vi "Data.vi"(8 "error in":errorcluster, 10 "Исходные данные":T1) -> (0 "error out":errorcluster)   [LabVIEW 2023, in "Initial Data.lvlib"]
doc: "_____\nCreated using DQMH Event Scripter 6.1.0.128."
uses:
  Initial Data.lvlib
  InitalData Type.ctl
  Data Argument--cluster.ctl
panel:
  # "Образец"
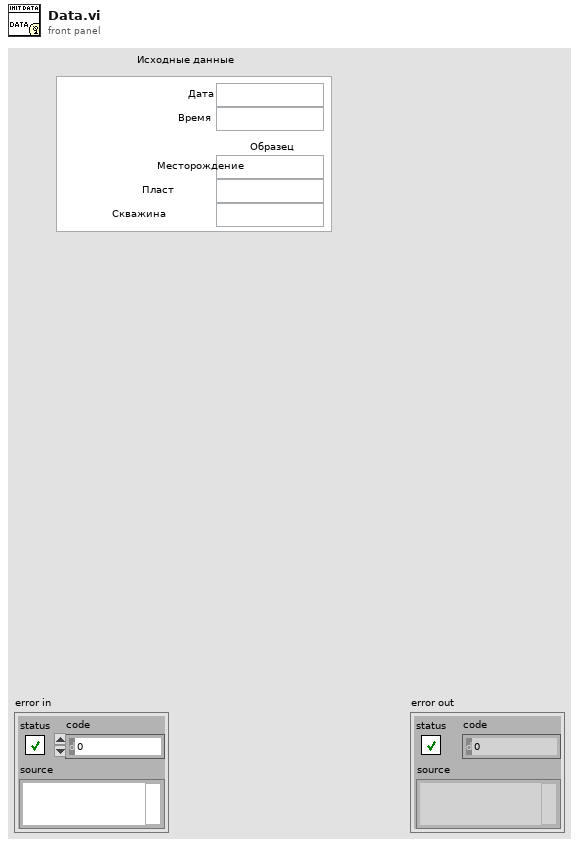
[diagram p1: front panel]
types:
  T1 = typedef "Initial Data.lvlib/InitalData Type.ctl" = cluster{"Дата":string, "Время":string, "Месторождение":string, "Пласт":string, "Скважина":string}
  T2 = typedef "Initial Data.lvlib/Data Argument--cluster.ctl" = cluster{"Исходные данные":T1}
  T3 = typedef "Initial Data.lvlib/Broadcast Events--cluster.ctl" = cluster{"Module Did Init":refnum<user-event>, "Status Updated":refnum<user-event>, "Error Reported":refnum<user-event>, "Module Did Stop":refnum<user-event>, "Update Module Execution Status":refnum<user-event>, "Data":refnum<user-event>}
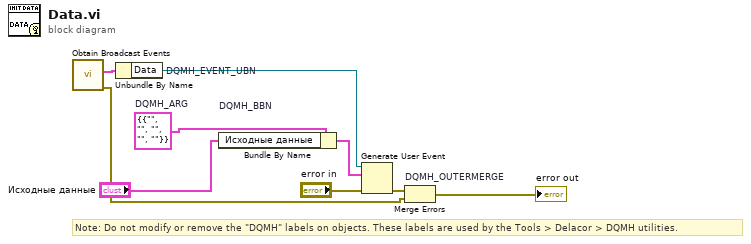
[diagram p0: block diagram]
diagram:
  w4 = T2 {"Исходные данные"={"Дата"="", "Время"="", "Месторождение"="", "Пласт"="", "Скважина"=""}}  # DQMH_ARG
  # "Note: Do not modify or remove the \"DQMH\" labels on objects. These labels are used by the Tools > Delacor > DQMH utilities."
  n1 = call "Obtain Broadcast Events.vi"() -> ("error out"=w2:errorcluster, "Initial Data Broadcast Events"=w1:T3)  [unwired: 10 in]
  n2 = Unbundle By Name "DQMH_EVENT_UBN"(w1) -> ("Data"=w6:refnum<user-event>)
  n3 = Bundle By Name "DQMH_BBN"(cluster=w4, "Исходные данные"="Исходные данные") -> (w7:T2)
  n4 = Generate User Event(user event=w6, event data cluster=w7, error in="error in") -> (error out=w5:errorcluster)  [unwired: 1 in, 1 out]
  n5 = Merge Errors "DQMH_OUTERMERGE"(w5, w2) -> (→"error out":errorcluster)
